vi "Get Image.vi"(8 "error in (no error)":errorcluster, 10 "Image":T1, 11 "CameraDevRef":T2={"Camera Address"="192.168.0.90", "CameraStatus"={"status"=FALSE, "code"=0, "source"=""}}) -> (0 "error out":errorcluster, 1 "Image Data String":string, 2 "Image Out":T1, 3 "CameraDevRef Out":T2)   [LabVIEW 2015]
doc: "Retrieves a specific image from the image data that the camera you specify acquired. Use the Start VI to start acquiring image data from the camera before you use the Get Image VI to retrieve an image. When you run this VI, this VI retrieves the most current snapshot of the image data from the camera.\n\nThis software is licensed. Open the labview\\readme\\WPI Robotics Library Open Source License.txt file for more information."
uses:
  <vilib>/Rock Robotics/WPI/Camera/WPI_CameraDevRef.ctl
  <vilib>/vision/Image Controls.llb/IMAQ Image.ctl
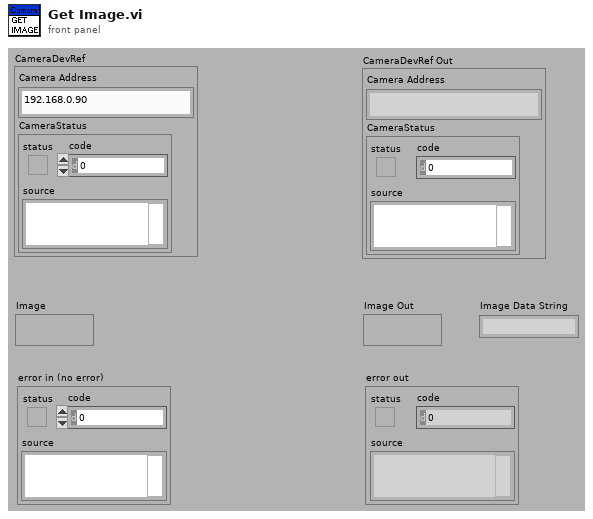
[diagram p1: front panel]
types:
  T1 = typedef "IMAQ Image.ctl" = refnum<image>
  T2 = typedef "WPI_CameraDevRef.ctl" = cluster{"Camera Address":string, "CameraStatus":errorcluster}
  T3 = enum16{"Update Mode", "Get Image", "Get Image Data"}
  T4 = typedef "WPI_CameraFrameRate.ctl" = u32
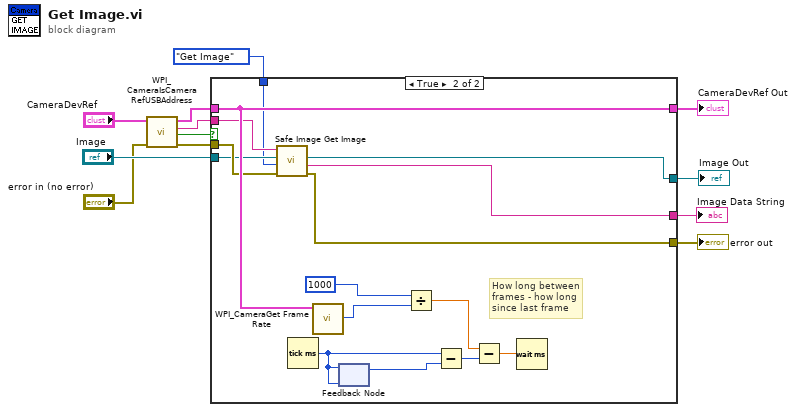
[diagram p0: block diagram]
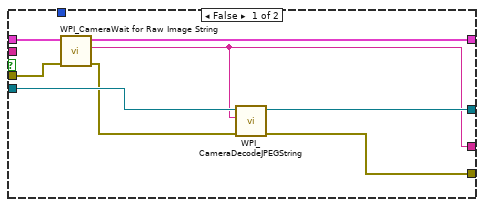
[diagram p2: hidden frame]
diagram:
  n1 = call <vilib>:"WPI_CameraIsCameraRefUSBAddress.vi"("error in (no error)"="error in (no error)", "CameraDevRef"="CameraDevRef") -> ("error out"=w7:errorcluster, "USB?"=w6:bool, "Camera Address Out"=w5:string, "CameraDevRef out"=w3:T2)  [unwired: 6 in]
  n2 = case shown="True" w6 {
    tunnel: "Image" -> [w20 w26]
    tunnel: [w19 w22] -> w11
    tunnel: [w18 w23] -> w10
    tunnel: w3 -> [w16 w31]
    tunnel: [w15 w31] -> w9
    tunnel: w5 -> [_ w25]
    tunnel: w7 -> [w14 w27]
    tunnel: T3."Get Image" ("Operation") -> [_ w24]
    tunnel: [w13 w21] -> w1
    frame False {
      n3 = call <vilib>:"WPI_CameraWait for Raw Image String.vi"("error in (no error)"=w14, "CameraDevRef"=w16) -> ("error out"=w17:errorcluster, "String"=w13:string, "CameraDevRef Out"=w15:T2)  [unwired: 3 in, 4 out]
      n4 = call <vilib>:"WPI_CameraDecodeJPEGString.vi"("error in"=w17, "Compressed Image"=w13, "Image In"=w20) -> ("error out"=w18:errorcluster, "Image Out"=w19:T1)  [unwired: 3 out]
    }
    frame True {
      # "How long between\nframes - how long\nsince last frame"
      n5 = call <vilib>:"Safe Image Get Image.vi"("error in"=w27, "Operation"=w24, "Image In"=w26, "Session In"=w25) -> ("error out"=w23:errorcluster, "Image Data String"=w21:string, "Image Out"=w22:T1)  [unwired: 4 in, 1 out]
      n6 = Tick Count (ms)() -> (millisecond timer value=w34:u32)
      n7 = call <vilib>:"WPI_CameraGet Frame Rate.vi"("CameraDevRef"=w31) -> ("Frame Rate (fps)"=w32:T4)  [unwired: 8 in, 2 out]
      n8 = feedback-in #1(w34) -> ()
      n9 = feedback #1(w34) -> (w35:u32)
      n10 = Divide(x=1000, y=w32) -> (x/y=w29:dbl)
      n11 = Subtract(x=w34, y=w35) -> (x-y=w30:u32)
      n12 = Subtract(x=w29, y=w30) -> (x-y=w28:dbl)
      n13 = Wait (ms)(milliseconds to wait=w28) -> ()  [unwired: 1 out]
    }
  }
  "CameraDevRef Out" <- w9
  "Image Out" <- w11
  "error out" <- w10
  "Image Data String" <- w1
